vi "readTagEPC.vi"(10 "Data Array":u8[](array[numeric]) format="%x") -> (2 "Freq":dbl format="%#.2g")   [LabVIEW 2018]
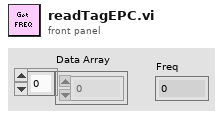
[diagram p1: front panel]
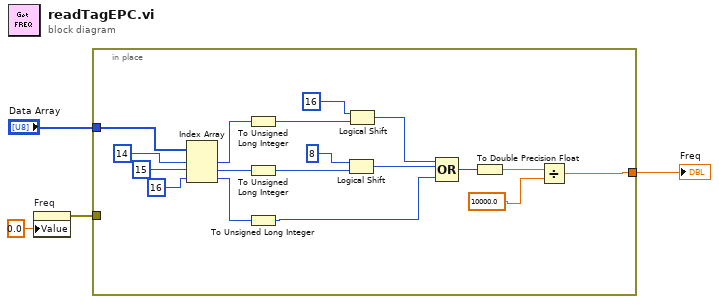
[diagram p0: block diagram]
diagram:
  n1 = property on="Freq" class="DigNum (strict)"("Value"=0.0 ("Freq")) -> (error out=w2:errorcluster)  [unwired: 2 in, 1 out]
  n2 = in-place {
    in-place-border: "Data Array" -> [w22]
    in-place-border: [w6] -> w3
    in-place-border: w2 -> [_]
    n3 = Index Array(array=w22, index #1=14 ("index"), index #2=15 ("index"), index #3=16 ("index")) -> (element #1=w18:u8, element #2=w17:u8, element #3=w16:u8)
    n4 = To Unsigned Long Integer(number=w18) -> (unsigned 32bit integer=w15:u32)
    n5 = To Unsigned Long Integer(number=w17) -> (unsigned 32bit integer=w14:u32)
    n6 = To Unsigned Long Integer(number=w16) -> (unsigned 32bit integer=w9:u32)
    n7 = Logical Shift(y=8, x=w14) -> (x << y=w10:u32)
    n8 = Logical Shift(y=16, x=w15) -> (x << y=w11:u32)
    n9 = Compound Arithmetic op=OR(w11, w10, w9) -> (w8:u32)
    n10 = To Double Precision Float(number=w8) -> (double precision float=w7:dbl)
    n11 = Divide(x=w7, y=10000.0) -> (x/y=w6:dbl)
  }
  "Freq" <- w3
